vi "Read States.vi"(8 "error in (no error)":errorcluster, 11 "ZigZagTactic in":refnum<class "ZigZagTactic.lvclass">) -> (0 "error out":errorcluster, 2 "States":enum16{"ZigZag", "Exit"}(ring), 3 "ZigZagTactic out":refnum<class "ZigZagTactic.lvclass">)   [LabVIEW 2023, in "ZigZagTactic.lvclass"]
uses:
  ZigZagTactic.lvclass
  ZigZagTactic.lvclass/ZigZagTactic.ctl
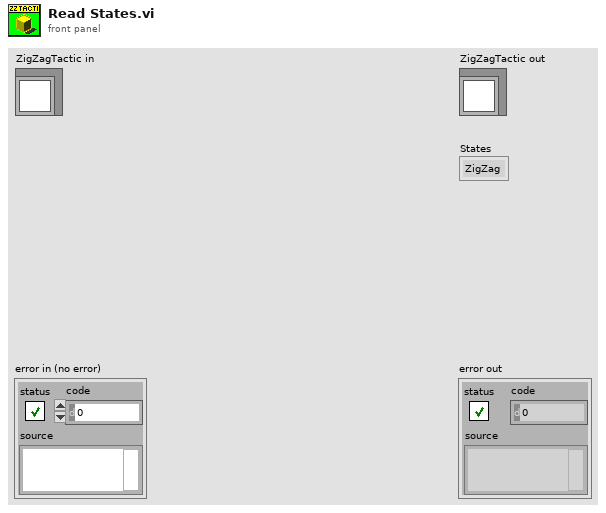
[diagram p1: front panel]
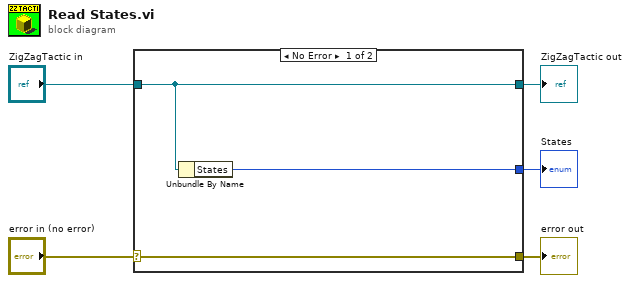
[diagram p0: block diagram]
diagram:
  n1 = case shown="No Error" "error in (no error)" {
    selector: "error in (no error)" -> [w8 w9]
    tunnel: [w8 w9] -> w4
    tunnel: [w7 w10] -> w2
    tunnel: "ZigZagTactic in" -> [w7 w10]
    tunnel: [w6 _] -> w1
    frame No Error {
      n2 = Unbundle By Name(w7) -> ("States"=w6:enum16{"ZigZag", "Exit"})
    }
    frame Error {
    }
  }
  "error out" <- w4
  "ZigZagTactic out" <- w2
  "States" <- w1
